vi "TranslateStatus.vi"(11 "Reply":string) -> (1 "Status":T1 {"Accel" scale=-2000.0..2000.0; "Position" scale=-100.0..100.0; "Gyro" scale=-1000.0..1000.0}, 3 "value":T2)   [LabVIEW 2020]
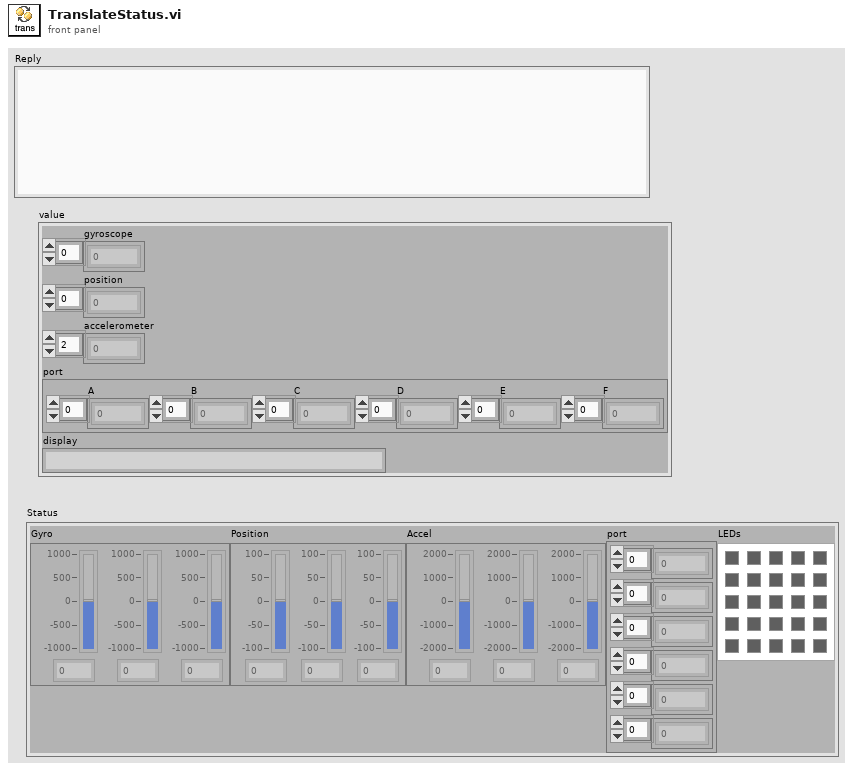
[diagram p1: front panel]
types:
  T1 = cluster{"Gyro":i32[], "Position":i32[], "Accel":i32[], "port":cluster{"A":i32[], "B":i32[], "C":i32[], "D":i32[], "E":i32[], "F":i32[]}, "LEDs":u32[][]}
  T2 = cluster{"gyroscope":i32[], "position":i32[], "accelerometer":i32[], "port":cluster{"A":i32[], "B":i32[], "C":i32[], "D":i32[], "E":i32[], "F":i32[]}, "display":string}
  T3 = cluster{"A":i32[], "B":i32[], "C":i32[], "D":i32[], "E":i32[], "F":i32[]}
  T4 = cluster{"gyroscope":i32[], "position":i32[], "accelerometer":i32[], "port":cluster{"A":i32[], "B":i32[], "C":i32[], "D":i32[], "E":i32[], "F":i32[]}, u32[][]}
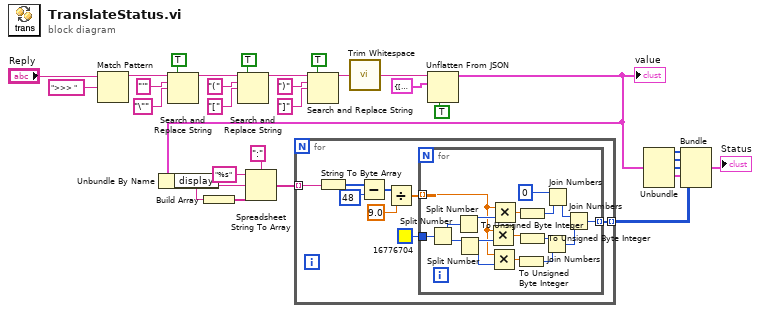
[diagram p0: block diagram]
diagram:
  n1 = Match Pattern(string="Reply", regular expression=">>> ") -> (before substring=w17:string)  [unwired: 1 in, 3 out]
  n2 = Search and Replace String(replace all?=TRUE ("ignore case? (F)"), input string=w17, search string="'", replace string="\"" ("replace string (\"\")")) -> (result string=w18:string)  [unwired: 4 in, 3 out]
  n3 = Search and Replace String(replace all?=TRUE ("ignore case? (F)"), input string=w18, search string="(", replace string="[" ("replace string (\"\")")) -> (result string=w24:string)  [unwired: 4 in, 3 out]
  n4 = Search and Replace String(replace all?=TRUE ("ignore case? (F)"), input string=w24, search string=")", replace string="]" ("replace string (\"\")")) -> (result string=w16:string)  [unwired: 4 in, 3 out]
  n5 = call <vilib>:"Trim Whitespace.vi"("string"=w16) -> ("trimmed string"=w13:string)  [unwired: 1 in]
  n6 = Unflatten From JSON(JSON string=w13, type and defaults=T2 {"gyroscope"=[], "position"=[], "accelerometer"=[], "port"={"A"=[], "B"=[], "C"=[], "D"=[], "E"=[], "F"=[]}, "display"=""}, default null elements? (F)=TRUE) -> (value=w7:T2)  [unwired: 4 in, 1 out]
  "value" <- w7
  n7 = Unbundle By Name(w7) -> ("display"=w10:string)
  n8 = Build Array(w10) -> (w11:string[])
  n9 = Spreadsheet String To Array(delimiter (Tab)=":", format string="%s", spreadsheet string=w10, array type (2D Dbl)=w11) -> (array=w8:string[])
  n10 = for {
    tunnel: w8 -> [w38] mode=indexing
    tunnel: [w32] -> w2 mode=indexing
    n11 = String To Byte Array(string=w38) -> (unsigned byte array=w37:u8[])
    n12 = Subtract(x=w37, y=48) -> (x-y=w35:i32[])
    n13 = Divide(x=w35, y=9.0) -> (x/y=w31:dbl[])
    n14 = for {
      tunnel: w31 -> [w49] mode=indexing
      tunnel: u32 16776704 ("Color Box") -> [w53]
      tunnel: [w46] -> w32 mode=indexing
      n15 = Split Number(x=w53) -> (hi(x)=w55:u16, lo(x)=w54:u16)
      n16 = Split Number(x=w55) -> (lo(x)=w51:u8)  [unwired: 1 out]
      n17 = Split Number(x=w54) -> (hi(x)=w50:u8, lo(x)=w52:u8)
      n18 = Multiply(x=w49, y=w50) -> (x*y=w42:dbl)
      n19 = Multiply(x=w49, y=w52) -> (x*y=w45:dbl)
      n20 = Multiply(x=w49, y=w51) -> (x*y=w41:dbl)
      n21 = To Unsigned Byte Integer(number=w45) -> (unsigned 8bit integer=w44:u8)
      n22 = To Unsigned Byte Integer(number=w41) -> (unsigned 8bit integer=w40:u8)
      n23 = To Unsigned Byte Integer(number=w42) -> (unsigned 8bit integer=w43:u8)
      n24 = Join Numbers(hi=w43, lo=w44) -> ((hi.lo)=w47:u16)
      n25 = Join Numbers(hi=u8 0, lo=w40) -> ((hi.lo)=w48:u16)
      n26 = Join Numbers(hi=w48, lo=w47) -> ((hi.lo)=w46:u32)
    }
  }
  n27 = Unbundle(w7) -> ("gyroscope"=w6:i32[], "position"=w4:i32[], "accelerometer"=w5:i32[], "port"=w3:T3)  [unwired: 1 out]
  n28 = Bundle("gyroscope"=w6, "position"=w4, "accelerometer"=w5, "port"=w3, w2) -> (→"Status":T4)  [unwired: 1 in]
